vi "TestCOMXYZandrootXYZ.vi"() -> ()   [LabVIEW 2012]
panel:
  in  "Z":dbl format="%#_13g"
  in  "Y":dbl format="%#_13g"
  in  "X":dbl format="%#_13g"
  out "XYZ":dbl
  out "CX":dbl
  in  "XYZandrootXYZ.IClass1":refnum<k7>
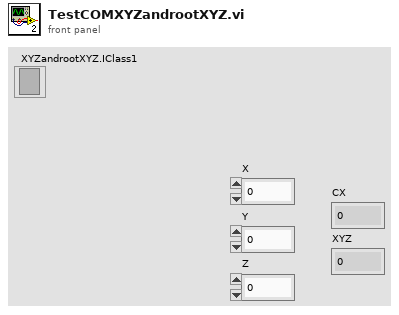
[diagram p1: front panel]
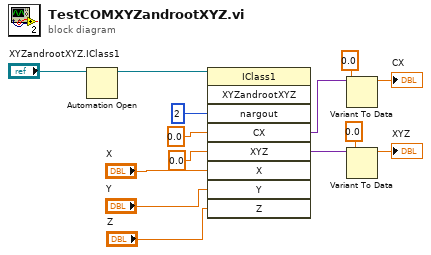
[diagram p0: block diagram]
diagram:
  n1 = Automation Open(Automation Refnum="XYZandrootXYZ.IClass1") -> (Automation Refnum=w13:refnum<k7>)  [unwired: 3 in, 1 out]
  n2 = invoke class="IClass1" method="XYZandrootXYZ"(reference=w13, "nargout"=2, "CX"=0.0, "XYZ"=0.0, "X"="X", "Y"="Y", "Z"="Z") -> ("CX"=w5:variant, "XYZ"=w4:variant)  [unwired: 2 in, 7 out]
  n3 = Variant To Data(type=0.0, Variant=w5) -> (data=→"CX":dbl)  [unwired: 1 in, 1 out]
  n4 = Variant To Data(type=0.0, Variant=w4) -> (data=→"XYZ":dbl)  [unwired: 1 in, 1 out]
